vi "Split multiple axes command.vi"(0 "System no.":i32=1 min=1 max=4 step=1, 1 "Command":T1(ring)=enum."POS?", 2 "Axes to command":string[](array[string]), 3 "Num. values in":dbl[](array[numeric]) format="%.6f", 4 "Bool. values in":bool[](array[boolean]), 5 "error in":errorcluster, 6 "Wait time (ms)":u32=10, 7 "No.of digits":i16=4, 11 "Stop refnum":refnum<vi>) -> (14 "Num. values out":dbl[](array[numeric]) format="%.6f", 15 "Bool. values out":bool[](array[boolean]), 19 "error out":errorcluster)   [LabVIEW 2026]
doc: "Splits command with more than one axis specification into the corresponding one-axis commands and returns answers for all given axes (if any). Wait time (ms) defines the time to wait between single commands. When using as a sub-VI, connect Stop refnum terminal to stop VI from caller. \nSupported commands are DCO, DCO?, MOV, MOV?, MVR, ONT?, OVF?, POS?, SVA, SVA?, SVO, SVO?, SVR, VOL? and General Wait for movement to stop (GWait)."
panel:
  in  "stop":bool
  # "Splits command with more than one axis specification into the corresponding one-axis commands and returns answers for all given axes (if any).  Wait time\ndefines the time to wait between single commands. When using as a sub-VI, connect Stop refnum terminal to stop VI from caller.  \nSupported commands are DCO, DCO?, MOV, MOV?, MVR, ONT?, OVF?, POS?, SVA, SVA?, SVO, SVO?, SVR, VOL? and General Wait for movement to stop (GWait)."
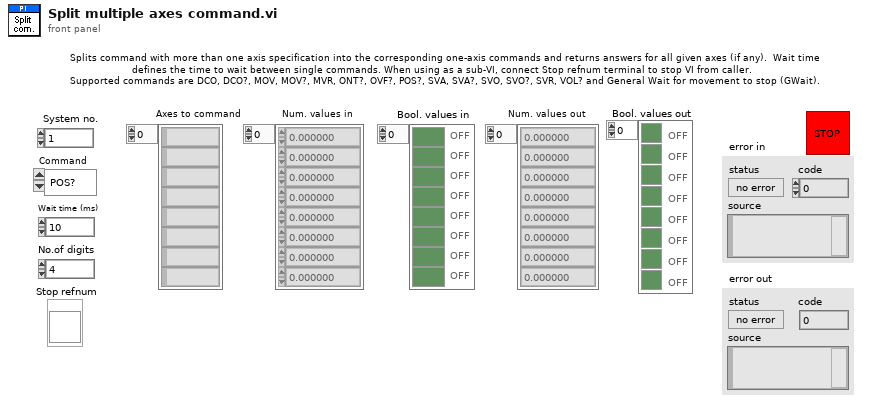
[diagram p1: front panel]
types:
  T1 = enum16{"DCO", "DCO?", "MOV", "MOV?", "MVR", "ONT?", "OVF?", "POS?", "RST", "SVA", "SVA?", "SVO", "SVO?", "SVR", "VOL?", "GWait"}
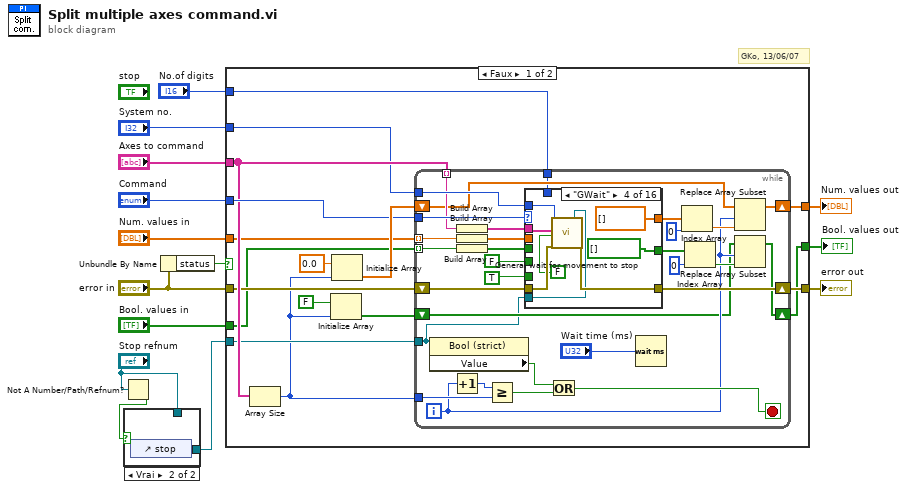
[diagram p0: block diagram]
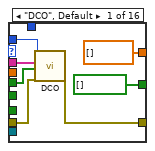
[diagram p3: hidden frame]
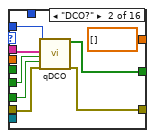
[diagram p4: hidden frame]
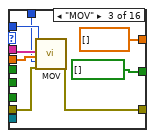
[diagram p5: hidden frame]
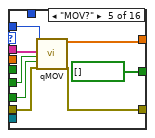
[diagram p6: hidden frame]
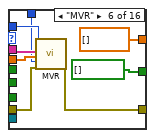
[diagram p7: hidden frame]
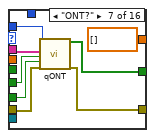
[diagram p8: hidden frame]
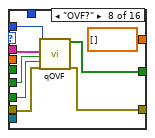
[diagram p9: hidden frame]
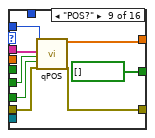
[diagram p10: hidden frame]
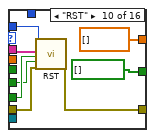
[diagram p11: hidden frame]
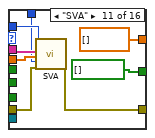
[diagram p12: hidden frame]
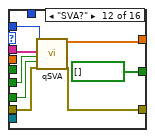
[diagram p13: hidden frame]
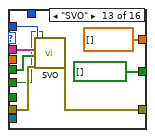
[diagram p14: hidden frame]
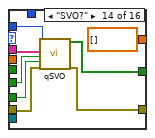
[diagram p15: hidden frame]
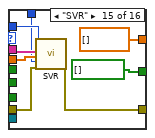
[diagram p16: hidden frame]
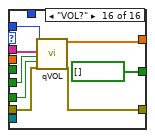
[diagram p17: hidden frame]
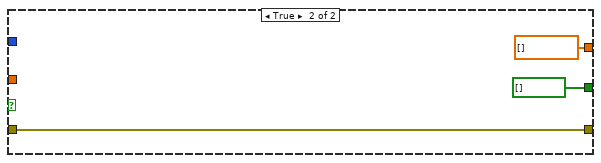
[diagram p18: hidden frame]
diagram:
  # "GKo, 13/06/07"
  n1 = Not A Number/Path/Refnum?(number/path/refnum="Stop refnum") -> (NaN/Path/Refnum?=w7:bool)
  n2 = case shown="Vrai" w7 {
    tunnel: [w15 w16] -> w5
    tunnel: "Stop refnum" -> [w15 _]
    frame False {
    }
    frame True {
      n3 = control-ref of="stop"() -> (w16:refnum<vi>)
    }
  }
  n4 = Unbundle By Name("error in") -> ("status"=w9:bool)
  n5 = case shown="Faux" w9 {
    tunnel: "Command" -> [w30 _]
    tunnel: "Axes to command" -> [w29 _]
    tunnel: "System no." -> [w28 _]
    tunnel: [w27 dbl[] []] -> w12
    tunnel: [w26 w193] -> w11
    tunnel: "error in" -> [w25 w193]
    tunnel: w5 -> [w24 _]
    tunnel: "Bool. values in" -> [w23 _]
    tunnel: "Num. values in" -> [w22 _]
    tunnel: [w18 bool[] []] -> w2
    tunnel: "No.of digits" -> [w17 _]
    frame False {
      n6 = Array Size(array=w29) -> (size(s)=w20:i32)
      n7 = Initialize Array(FALSE, w20) -> (w19:bool[])
      n8 = Initialize Array(0.0, w20) -> (w31:dbl[])
      n9 = while {
        tunnel: w29 -> [w57] mode=indexing
        tunnel: w28 -> [w63]
        shift-right: [w59] -> w27
        shift-left: w31 -> [w41]
        tunnel: w30 -> [w58]
        shift-right: [w53] -> w26
        shift-left: w25 -> [w52]
        tunnel: w24 -> [w33]
        tunnel: w20 -> [w49]
        tunnel: w23 -> [w47] mode=indexing
        tunnel: w22 -> [w44] mode=indexing
        shift-right: [w36] -> w18
        shift-left: w19 -> [w39]
        tunnel: w17 -> [w35]
        i -> [w40]
        stop <- w48 stop-if-true
        n10 = property class="Bool (strict)"(reference=w33) -> ("Value"=w50:bool)  [unwired: 1 in, 2 out]
        n11 = Increment(x=w40) -> (x+1=w34:i32)
        n12 = Build Array(w57) -> (w62:string[])
        n13 = Build Array(w44) -> (w45:dbl[])
        n14 = Build Array(w47) -> (w46:bool[])
        n15 = Greater Or Equal?(x=w34, y=w49) -> (x >= y?=w51:bool)
        n16 = case shown="\"GWait\"" w58 {
          tunnel: w52 -> [w70 w76 w84 w92 w100 w108 w116 w124 w132 w140 w148 w156 w166 w172 w180 w188]
          tunnel: w63 -> [w69 w78 w86 w94 w102 w110 w118 w126 w134 w142 w150 w158 w165 w174 w182 w190]
          tunnel: [w68 w75 w83 w91 w99 w107 w115 w123 w131 w139 w147 w155 w164 w171 w179 w187] -> w53
          tunnel: w62 -> [w67 w77 w85 w93 w101 w109 w117 w125 w133 w141 w149 w157 w163 w173 w181 w189]
          tunnel: [dbl[] [] dbl[] [] ("Position") dbl[] [] ("Position") dbl[] [] ("Position") w98 dbl[] [] ("Position") dbl[] [] ("Position") dbl[] [] ("Position") w130 dbl[] [] ("Position") dbl[] [] ("Position") w154 dbl[] [] dbl[] [] ("Position") dbl[] [] ("Position") w186] -> w61
          tunnel: FALSE ("All axes?") -> [_ w74 _ _ w97 _ w114 w122 w129 w135 _ w153 w159 w170 _ w185]
          tunnel: TRUE ("Axis identifier?") -> [_ w73 _ _ w96 _ w113 w121 w128 w136 _ w152 _ w169 _ w184]
          tunnel: w46 -> [w65 _ _ _ _ _ _ _ _ _ _ _ w161 _ _ _]
          tunnel: w45 -> [_ _ w80 _ _ w104 _ _ _ _ w144 _ _ _ w176 _]
          tunnel: [bool[] [] ("Drift comp. mode?") w72 bool[] [] ("Drift comp. mode?") bool[] [] ("Drift comp. mode?") bool[] [] ("Drift comp. mode?") bool[] [] ("Drift comp. mode?") w112 w120 bool[] [] ("Drift comp. mode?") bool[] [] ("Drift comp. mode?") bool[] [] ("Drift comp. mode?") bool[] [] ("Drift comp. mode?") bool[] [] ("Drift comp. mode?") w168 bool[] [] ("Drift comp. mode?") bool[] [] ("Drift comp. mode?")] -> w38
          tunnel: w35 -> [_ _ w79 _ _ w103 _ _ _ _ w143 _ _ _ w175 _]
          tunnel: w33 -> [_ _ _ w87 _ _ _ _ _ _ _ _ _ _ _ _]
          frame "DCO", Default {
            n17 = call "DCO.vi"("System no."=w69, "Axes to command"=w67, "Drift comp. mode"=w65, "error in"=w70) -> ("error out"=w68:errorcluster)  [unwired: 1 in, 14 out]
          }
          frame "DCO?" {
            n18 = call "qDCO.vi"("System no."=w78, "Axes to query"=w77, "All axes?"=w74, "Axis identifier?"=w73, "error in"=w76) -> ("Drift comp. mode?"=w72:bool[], "error out"=w75:errorcluster)  [unwired: 13 out]
          }
          frame "MOV" {
            n19 = call "MOV.vi"("System no."=w86, "Axes to move"=w85, "Position values"=w80, "No.of digits"=w79, "error in"=w84) -> ("error out"=w83:errorcluster)  [unwired: 14 out]
          }
          frame "GWait" {
            n20 = call "General wait for movement to stop.vi"("System no."=w94, "Axes to wait for"=w93, "All axes?"=FALSE, "error in"=w92, "Stop refnum"=w87) -> ("error out"=w91:errorcluster)  [unwired: 3 in, 11 out]
          }
          frame "MOV?" {
            n21 = call "qMOV.vi"("System no."=w102, "Axes to query"=w101, "All axes?"=w97, "Axis identifier?"=w96, "error in"=w100) -> ("Target position"=w98:dbl[], "error out"=w99:errorcluster)  [unwired: 13 out]
          }
          frame "MVR" {
            n22 = call "MVR.vi"("System no."=w110, "Axes to move"=w109, "Position values"=w104, "No.of digits"=w103, "error in"=w108) -> ("error out"=w107:errorcluster)  [unwired: 14 out]
          }
          frame "ONT?" {
            n23 = call "qONT.vi"("System no."=w118, "Axes to query"=w117, "All axes?"=w114, "Axis identifier?"=w113, "error in"=w116) -> ("Axis on target?"=w112:bool[], "error out"=w115:errorcluster)  [unwired: 13 out]
          }
          frame "OVF?" {
            n24 = call "qOVF.vi"("System no."=w126, "Axes to query"=w125, "All axes?"=w122, "Axis identifier?"=w121, "error in"=w124) -> ("Axis overflow?"=w120:bool[], "error out"=w123:errorcluster)  [unwired: 13 out]
          }
          frame "POS?" {
            n25 = call "qPOS.vi"("System no."=w134, "Axes to query"=w133, "All axes?"=w129, "Axis identifier?"=w128, "error in"=w132) -> ("Position"=w130:dbl[], "error out"=w131:errorcluster)  [unwired: 13 out]
          }
          frame "RST" {
            n26 = call "RST.vi"("System no."=w142, "Axes to be restored"=w141, "All axes?"=w136, "Axis identifier?"=w135, "error in"=w140) -> ("error out"=w139:errorcluster)  [unwired: 14 out]
          }
          frame "SVA" {
            n27 = call "SVA.vi"("System no."=w150, "Axes to move"=w149, "PZT voltage"=w144, "No.of digits"=w143, "error in"=w148) -> ("error out"=w147:errorcluster)  [unwired: 14 out]
          }
          frame "SVA?" {
            n28 = call "qSVA.vi"("System no."=w158, "Axes to query"=w157, "All axes?"=w153, "Axis identifier?"=w152, "error in"=w156) -> ("Commanded PZT voltage"=w154:dbl[], "error out"=w155:errorcluster)  [unwired: 13 out]
          }
          frame "SVO" {
            n29 = call "SVO.vi"("System no."=w165, "Axes to command"=w163, "Servo mode"=w161, "error in"=w166, "Without axis ID?"=w159) -> ("error out"=w164:errorcluster)  [unwired: 14 out]
          }
          frame "SVO?" {
            n30 = call "qSVO.vi"("System no."=w174, "Axes to query"=w173, "All axes?"=w170, "Axis identifier?"=w169, "error in"=w172) -> ("Servo status?"=w168:bool[], "error out"=w171:errorcluster)  [unwired: 13 out]
          }
          frame "SVR" {
            n31 = call "SVR.vi"("System no."=w182, "Axes to move"=w181, "PZT voltage"=w176, "No.of digits"=w175, "error in"=w180) -> ("error out"=w179:errorcluster)  [unwired: 14 out]
          }
          frame "VOL?" {
            n32 = call "qVOL.vi"("System no."=w190, "Axes to query"=w189, "All axes?"=w185, "Axis identifier?"=w184, "error in"=w188) -> ("Current PZT voltage"=w186:dbl[], "error out"=w187:errorcluster)  [unwired: 13 out]
          }
        }
        n33 = Or(x=w50, y=w51) -> (x .or. y?=w48:bool)
        n34 = Wait (ms)(milliseconds to wait="Wait time (ms)") -> ()  [unwired: 1 out]
        n35 = Index Array(array=w61, index=0 ("Index")) -> (element=w60:dbl)
        n36 = Index Array(array=w38, index=0 ("Index")) -> (element=w42:bool)
        n37 = Replace Array Subset(array=w41, new element=w60, index=w40) -> (w59:dbl[])
        n38 = Replace Array Subset(array=w39, new element=w42, index=w40) -> (w36:bool[])
      }
    }
    frame True {
    }
  }
  "error out" <- w11
  "Num. values out" <- w12
  "Bool. values out" <- w2
